vi "Double Functional Global.vi"(10 "Action":enum16{"Get Data", "Set Data"}(ring), 11 "Input":dbl) -> (3 "Output":dbl)   [LabVIEW 2014]
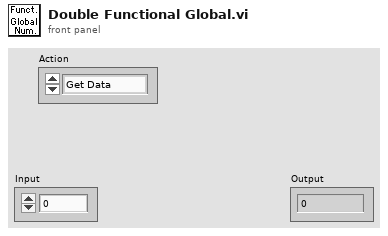
[diagram p1: front panel]
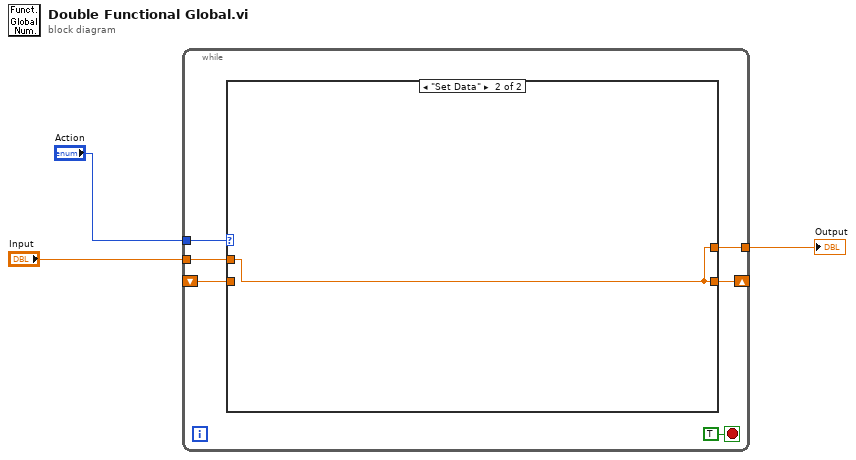
[diagram p0: block diagram]
diagram:
  n1 = while {
    tunnel: "Action" -> [w8]
    shift-right: [w6] -> _
    shift-left: _ -> [w5]
    tunnel: "Input" -> [w7]
    tunnel: [w4] -> w1
    stop <- TRUE stop-if-true
    n2 = case shown="\"Set Data\"" w8 {
      tunnel: w7 -> [_ w11]
      tunnel: [w10 w11] -> w6
      tunnel: w5 -> [w10 _]
      tunnel: [w10 w11] -> w4
      frame "Get Data", Default {
      }
      frame "Set Data" {
      }
    }
  }
  "Output" <- w1
